vi "test-diff2.vi"() -> ()   [LabVIEW 2021]
panel:
  in  "Numeric 3":dbl
  out "Numeric 2":dbl
  in  "Numeric":dbl
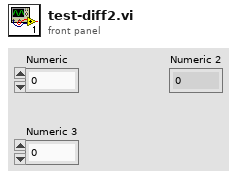
[diagram p1: front panel]
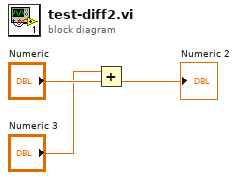
[diagram p0: block diagram]
diagram:
  n1 = Add(x="Numeric 3", y="Numeric") -> (x+y=→"Numeric 2":dbl)
